vi "set max exposure time.vi"(8 "error in (no error)":errorcluster, 11 "Thorcam in":refnum<class "Thorcam.lvclass">) -> (0 "error out":errorcluster, 3 "Thorcam out":refnum<class "Thorcam.lvclass">)   [LabVIEW 2012, in "Thorcam.lvclass"]
uses:
  Thorcam.lvclass
  Thorcam.lvclass/Thorcam.ctl
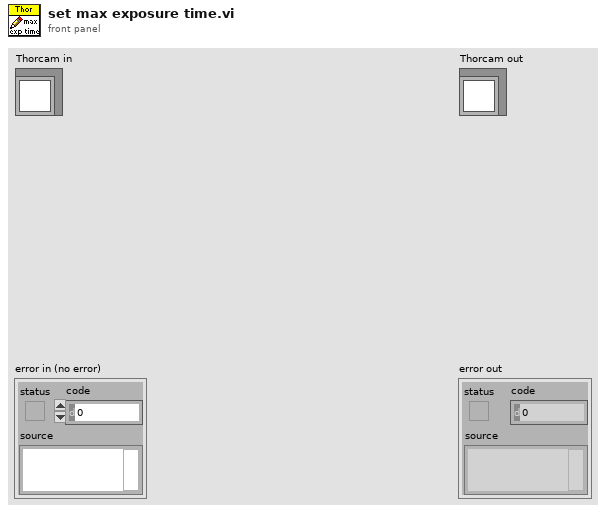
[diagram p1: front panel]
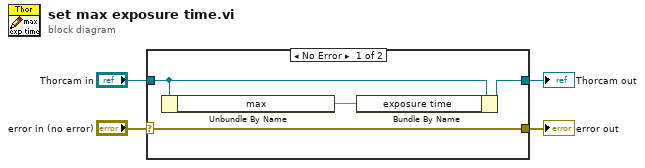
[diagram p0: block diagram]
diagram:
  n1 = case shown="No Error" "error in (no error)" {
    selector: "error in (no error)" -> [w8 w10]
    tunnel: [w8 w10] -> w3
    tunnel: [w5 w9] -> w1
    tunnel: "Thorcam in" -> [w6 w9]
    frame No Error {
      n2 = Unbundle By Name(w6) -> ("max"=w7:dbl[unit])
      n3 = Bundle By Name(cluster=w6, "exposure time"=w7) -> (w5:refnum<class "Thorcam.lvclass">)
    }
    frame Error {
    }
  }
  "error out" <- w3
  "Thorcam out" <- w1
